vi "SbigQueryImage.vi"(3 "Sbig":string="PI1-SBIG", 9 "error in (no error)":errorcluster) -> (0 "Sbig out":string="PI1-SBIG", 2 "Image":i32[][](graph), 6 "error out":errorcluster)   [LabVIEW 2009]
uses:
  Controls/SbigStatus.ctl
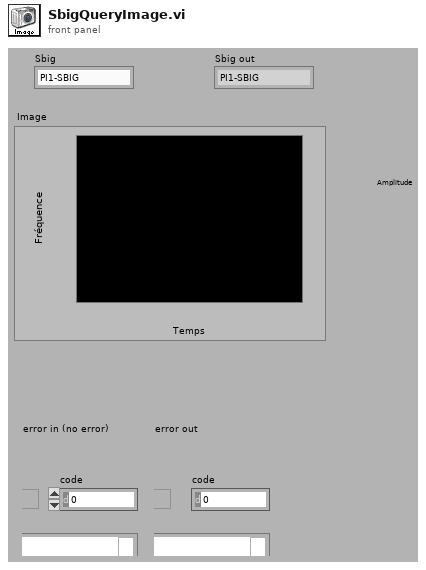
[diagram p1: front panel]
types:
  T1 = typedef "SbigStatus.ctl" = cluster{"Managed ?":bool, "State":enum16{"IDLE", "EXPOSING", "READING"}, "Image":i32[][], "Temperature Info":cluster{"Temperature Regulation":bool, "T Setpoint":dbl, "T CCD":dbl, "T Ambient":dbl, "Cooling %":dbl}}
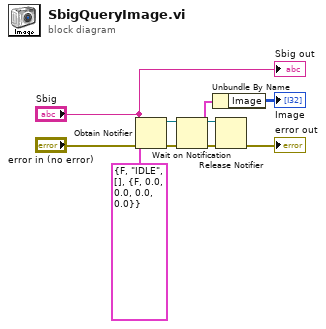
[diagram p0: block diagram]
diagram:
  n1 = Obtain Notifier(name (unnamed)="Sbig", notification data type=T1 {"Managed ?"=FALSE, "State"=enum."IDLE", "Image"=[], "Temperature Info"={"Temperature Regulation"=FALSE, "T Setpoint"=0.0, "T CCD"=0.0, "T Ambient"=0.0, "Cooling %"=0.0}} ("SbigStatus"), error in (no error)="error in (no error)") -> (notifier out=w6:refnum<notifier>, error out=w7:errorcluster)  [unwired: 1 in, 1 out]
  n2 = Wait on Notification(notifier=w6, error in (no error)=w7) -> (notifier out=w9:refnum<notifier>, notification=w2:T1, error out=w8:errorcluster)  [unwired: 3 out]
  n3 = Unbundle By Name(w2) -> ("Image"=→"Image":i32[][])
  n4 = Release Notifier(notifier=w9, error in (no error)=w8) -> (error out=→"error out":errorcluster)  [unwired: 3 out]
  "Sbig out" <- "Sbig"
